vi "PCM Vertical Panel.vi"() -> ()   [LabVIEW 2016, in "PCM PanelSplit.lvclass"]
uses:
  PCM PanelSplit.lvclass
  PanelSplitToolkit/PanelObject/PanelObject.lvclass
  <vilib>/Utility/error.llb/DialogType.ctl
  PanelSplitToolkit/QueueManager.llb/CreatQueue.vi
  PanelSplitToolkit/QueueManager.llb/Remove.vi
  PanelSplitToolkit/QueueManager.llb/Destroy.vi
  PanelSplitToolkit/QueueManager.llb/Insert.vi
  PanelSplitToolkit/PanelDataNode/PanelDataNode.lvclass
  PanelSplitToolkit/PanelDataNode/Split Mode.ctl
panel:
  in  "Node*":refnum<data-value>
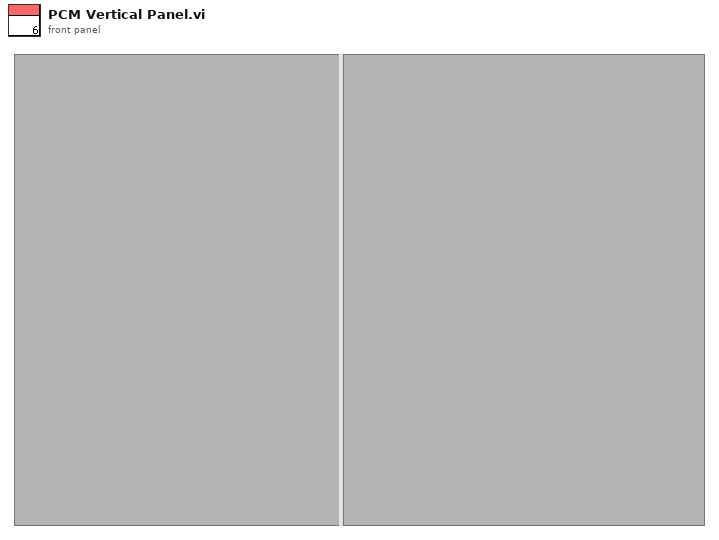
[diagram p1: front panel]
types:
  T1 = cluster{"error":errorcluster, "Event":string, "Data":variant, "Q_Local":string, "Caller":string}
  T2 = typedef "PanelDataNode.lvclass/Split Mode.ctl" = enum16{"Horizontal(up)", "Vertical(left)", "Horizontal(down)", "Vertical(right)"}
  T3 = typedef "DialogType.ctl" = u16
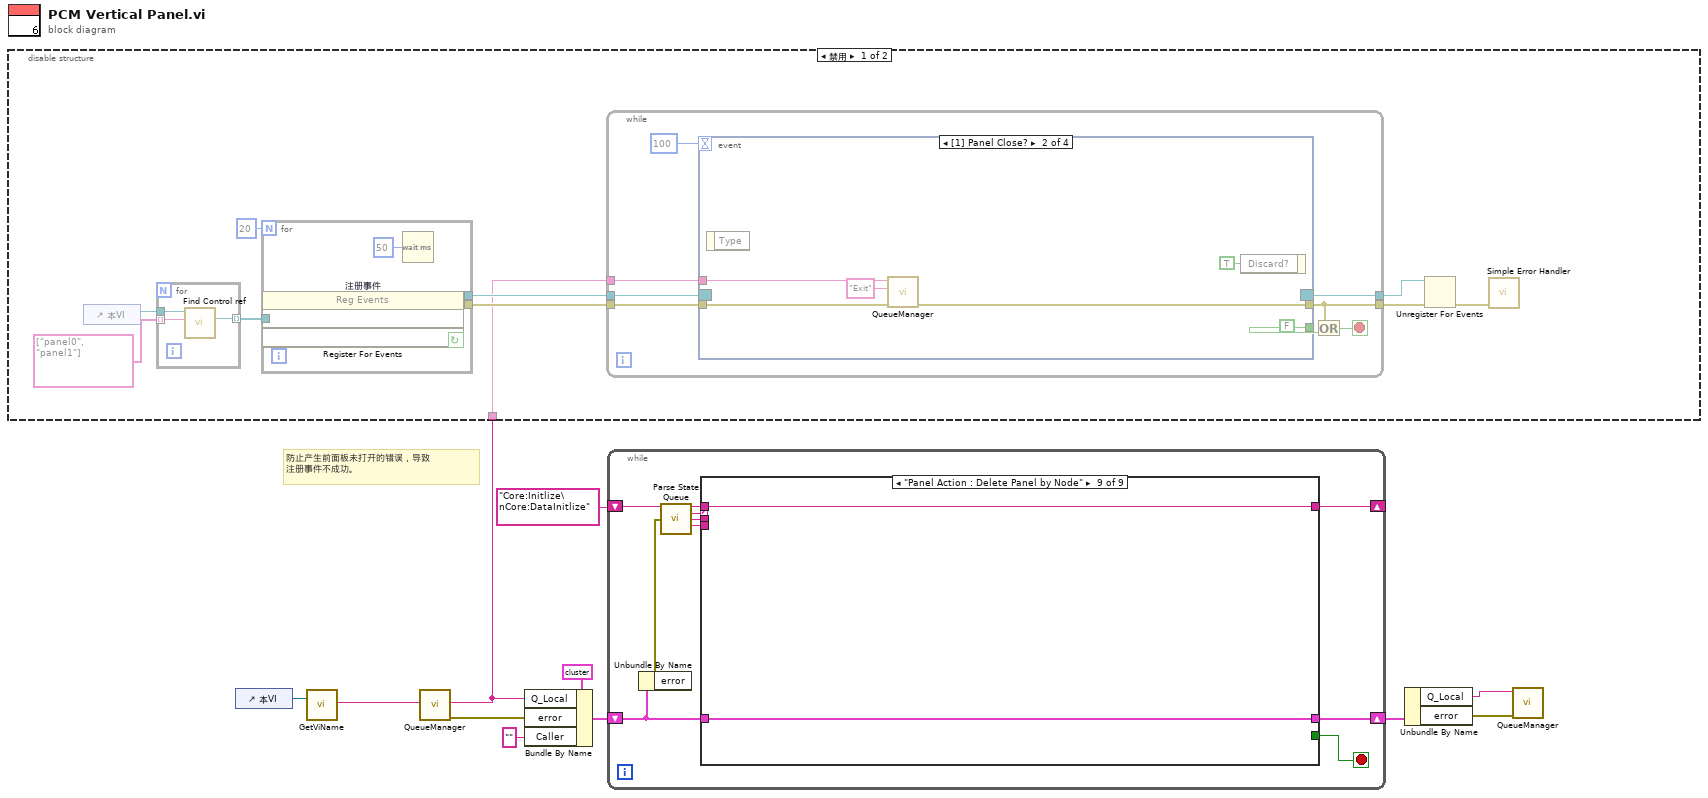
[diagram p0: block diagram]
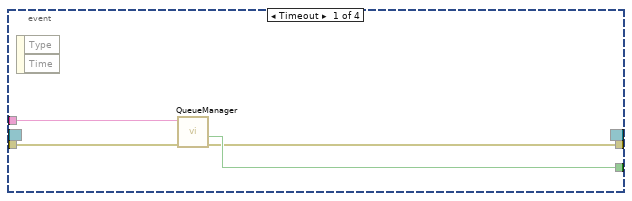
[diagram p2: hidden frame]
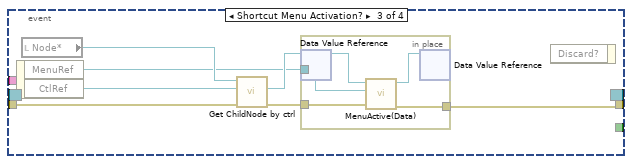
[diagram p3: hidden frame]
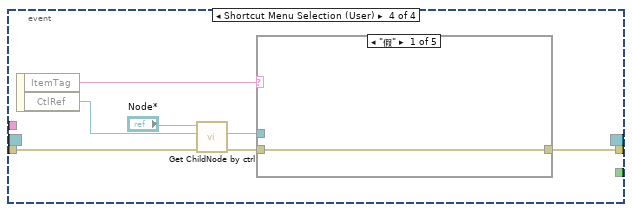
[diagram p4: hidden frame]
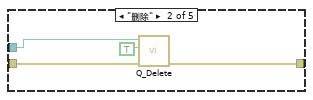
[diagram p5: hidden frame]
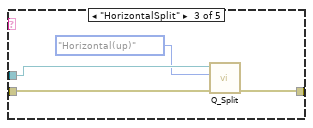
[diagram p6: hidden frame]
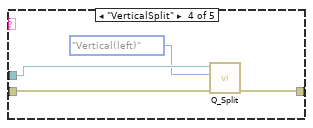
[diagram p7: hidden frame]
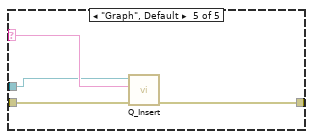
[diagram p8: hidden frame]
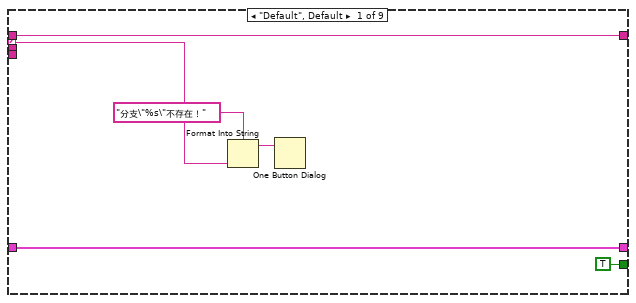
[diagram p10: hidden frame]
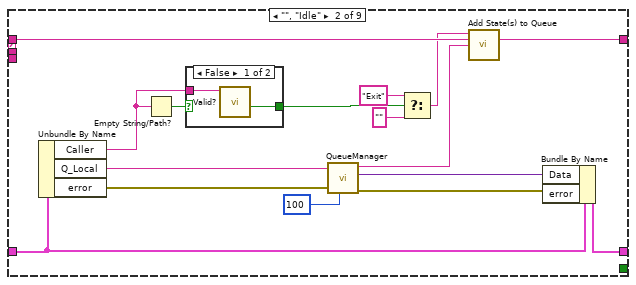
[diagram p11: hidden frame]
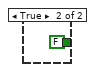
[diagram p12: hidden frame]
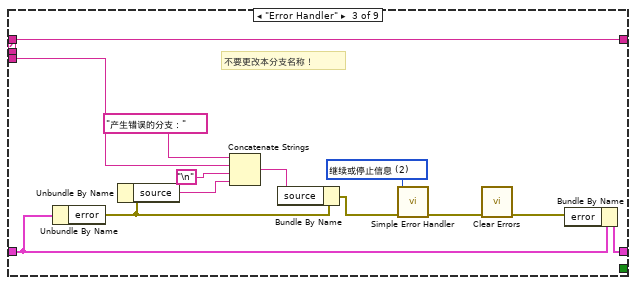
[diagram p13: hidden frame]
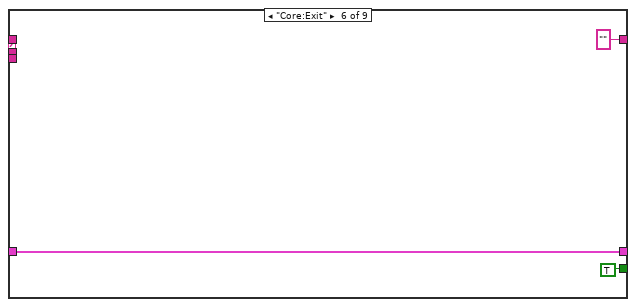
[diagram p16: hidden frame]
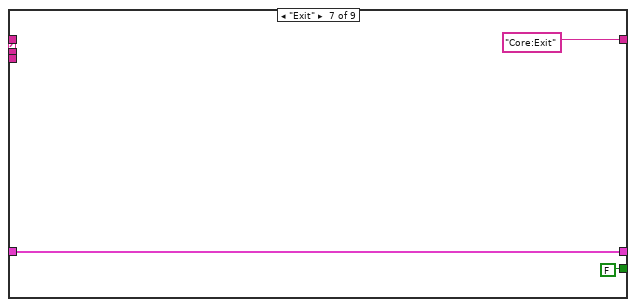
[diagram p17: hidden frame]
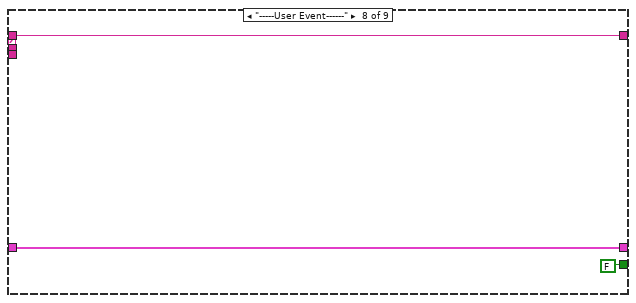
[diagram p18: hidden frame]
diagram:
  # "防止产生前面板未打开的错误，导致\n注册事件不成功。"
  n1 = control-ref of="本VI"() -> (w3:refnum<vi>)
  n2 = call "GetViName.vi"("VI*"=w3) -> ("VI Name"=w1:string)  [unwired: 9 in, 1 out]
  n3 = disable-structure shown="禁用" {
    disable-tunnel: w1 -> [w18 _]
    frame Disabled {
      n4 = control-ref of="本VI"() -> (w12:refnum<vi>)
      n5 = for {
        tunnel: w12 -> [w23]
        tunnel: string[] ["panel0", "panel1"] -> [w22] mode=indexing
        tunnel: [w21] -> w17 mode=indexing
        n6 = call "Find Control ref.vi"("control name"=w22, "panelvi*"=w23) -> ("ctrl*"=w21:refnum<vi>)  [unwired: 7 in, 2 out]
      }
      n7 = for {
        N: 20 -> [_]
        tunnel: [w25] -> w20
        tunnel: [w27] -> w19
        tunnel: w17 -> [w26]
        stop <- w25 continue-if-true
        n8 = register-events "注册事件"(w26, w26) -> (reference out=w27:refnum<event-registration>, error out=w25:errorcluster)  [unwired: 2 in]
        n9 = Wait (ms)(milliseconds to wait=u32 50 ("等待时间（毫秒）")) -> ()  [unwired: 1 out]
      }
      n10 = while {
        tunnel: w20 -> [w29]
        tunnel: w18 -> [w35]
        tunnel: [w32] -> w15
        tunnel: w19 -> [w30]
        tunnel: [w28] -> w13
        stop <- w33 stop-if-true
        n11 = event shown="[1] Panel Close?" {
          selector: w30 -> [_ _ _ _]
          dyn-events: [_ _ _ _] -> w28
          timeout: 100 -> [_ _ _ _]
          tunnel: [w37 FALSE _ _] -> w34
          tunnel: w35 -> [w39 w44 _ _]
          tunnel: w29 -> [w38 w43 w49 w62]
          tunnel: [w36 w42 w47 w60] -> w32
          event Timeout {
            n12 = event-data() -> ()  [unwired: 1 in, 2 out]
            n13 = call-poly "QueueManager.vi"("error in (no error)"=w38, "Queue Name(unamed)"=w39) -> ("error out"=w36:errorcluster, "Not Exist?"=w37:bool)  [unwired: 8 in]
          }
          event Panel Close? {
            n14 = event-data() -> ()  [unwired: 1 in, 1 out]
            n15 = call-poly "QueueManager.vi"("error in"=w43, "Event"="Exit", "QueueName"=w44) -> ("error out"=w42:errorcluster)  [unwired: 7 in, 1 out]
            n16 = event-data("Discard?"=TRUE ("放弃？")) -> ()  [unwired: 1 in, 1 out]
          }
          event Shortcut Menu Activation? {
            n17 = event-data() -> ("MenuRef"=w46:refnum<k9>, "CtlRef"=w50:refnum<vi>)  [unwired: 1 in]
            n18 = local read "Node*"() -> (w51:refnum<data-value>)
            n19 = call "Get ChildNode by ctrl.vi"("error in (no error)"=w49, "ctr*"=w50, "Node*"=w51) -> ("error out"=w48:errorcluster, "ChildNode*"=w52:refnum<data-value>)  [unwired: 7 in]
            n20 = in-place {
              in-place-border: w46 -> [w56]
              in-place-border: w48 -> [w54]
              in-place-border: [w53] -> w47
              n21 = in-place-dvr #1(w52) -> (w57:refnum<class "PanelDataNode.lvclass">)  [unwired: 1 out]
              n22 = call-dynamic "MenuActive(Data).vi"("error in"=w54, "Menu Reference in"=w56, "PanelDataNode in"=w57) -> ("error out"=w53:errorcluster, "PanelDataNode out"=w55:refnum<class "PanelDataNode.lvclass">)  [unwired: 6 in, 1 out]
              n23 = in-place-dvr #1(w55) -> ()  [unwired: 2 out]
            }
            n24 = event-data() -> ()  [unwired: 2 in, 1 out]
          }
          event Shortcut Menu Selection (User) {
            n25 = event-data() -> ("ItemTag"=w59:string, "CtlRef"=w63:refnum<vi>)  [unwired: 1 in]
            n26 = call "Get ChildNode by ctrl.vi"("error in (no error)"=w62, "ctr*"=w63, "Node*"="Node*") -> ("error out"=w61:errorcluster, "ChildNode*"=w58:refnum<data-value>)  [unwired: 7 in]
            n27 = case shown="\"假\"" w59 {
              selector: w59 -> [_ _ _ _ w81]
              tunnel: w61 -> [w65 w68 w73 w77 w80]
              tunnel: [w65 w67 w72 w76 w78] -> w60
              tunnel: w58 -> [_ w66 w71 w75 w79]
              frame "假" {
              }
              frame "删除" {
                n28 = call "Q_Delete.vi"("error in"=w68, "CloseVI?(T)"=TRUE, "ChildNode*"=w66) -> ("error out"=w67:errorcluster)  [unwired: 8 in]
              }
              frame "HorizontalSplit" {
                n29 = call "Q_Split.vi"("error in"=w73, "Split Mode"=Split_Mode."Horizontal(up)", "ChildNode*"=w71) -> ("error out"=w72:errorcluster)  [unwired: 8 in]
              }
              frame "VerticalSplit" {
                n30 = call "Q_Split.vi"("error in"=w77, "Split Mode"=Split_Mode."Vertical(left)", "ChildNode*"=w75) -> ("error out"=w76:errorcluster)  [unwired: 8 in]
              }
              frame "Graph", Default {
                n31 = call "Q_Insert.vi"("error in"=w80, "Vi Alias"=w81, "ChildNode*"=w79) -> ("error out"=w78:errorcluster)  [unwired: 8 in]
              }
            }
          }
        }
        n32 = Or(x=w32, y=w34) -> (x .or. y?=w33:bool)
      }
      n33 = Unregister For Events(event registration refnum=w13, error in=w15) -> (error out=w14:errorcluster)
      n34 = call <vilib>:"Simple Error Handler.vi"("error in (no error)"=w14) -> ()  [unwired: 4 in, 5 out]
    }
    frame Enabled {
    }
  }
  n35 = call-poly "QueueManager.vi"("QueueName"=w1) -> ("error out"=w2:errorcluster)  [unwired: 9 in, 1 out]
  n36 = Bundle By Name(cluster=T1 {"error"={"status"=FALSE, "code"=0, "source"=""}, "Event"="", "Data"=variant, "Q_Local"="", "Caller"=""} ("TmpData"), "Q_Local"=w1, "error"=w2, "Caller"="") -> (w6:T1)
  n37 = while {
    shift-right: [w85] -> w8
    shift-left: w6 -> [w86]
    shift-right: [w84] -> _
    shift-left: "Core:Initlize\nCore:DataInitlize" -> [w91]
    stop <- w88 stop-if-true
    n38 = Unbundle By Name(w86) -> ("error"=w87:errorcluster)
    n39 = call "Parse State Queue.vi"("State Queue"=w91, "Error In (no error)"=w87) -> ("Remaining States"=w90:string, "Current State"=w89:string, "Arguments"=w83:string, "PreState"=w82:string)  [unwired: 10 in]
    n40 = case shown="\"Panel Action : Delete Panel by Node\"" w89 {
      selector: w89 -> [w95 _ _ _ _ _ _ _ _]
      tunnel: w90 -> [w96 w110 w129 w131 w133 _ _ w140 w143]
      tunnel: w83 -> [_ _ _ _ _ _ _ _ _]
      tunnel: [TRUE _ _ _ _ TRUE FALSE FALSE _] -> w88
      tunnel: w86 -> [w97 w107 w126 w130 w132 w135 w138 w141 w144]
      tunnel: [w97 w112 w125 w130 w132 w135 w138 w141 w144] -> w85
      tunnel: [w96 w109 w129 w131 w133 "" ("Remaining States") "Core:Exit" ("Remaining States") w140 w143] -> w84
      tunnel: w82 -> [_ _ w123 _ _ _ _ _ _]
      frame "Default", Default {
        n41 = Format Into String(format string="分支\"%s\"不存在！" ("格式字符串"), w95) -> (resulting string=w94:string)  [unwired: 2 in, 1 out]
        n42 = One Button Dialog(message=w94) -> ()  [unwired: 1 in, 1 out]
      }
      frame "", "Idle" {
        n43 = Unbundle By Name(w107) -> ("Caller"=w101:string, "Q_Local"=w106:string, "error"=w105:errorcluster)
        n44 = Empty String/Path?(string/path=w101) -> (empty?=w104:bool)
        n45 = case shown="False" w104 {
          tunnel: [w115 FALSE ("Not Exist?")] -> w103
          tunnel: w101 -> [w114 _]
          frame False {
            n46 = call "Valid?.vi"("Queue Name(unamed)"=w114) -> ("Not Exist?"=w115:bool)  [unwired: 9 in, 1 out]
          }
          frame True {
          }
        }
        n47 = call-poly "QueueManager.vi"("Time out(-1)"=100, "error in (no error)"=w105, "Queue Name"=w106) -> ("error out"=w113:errorcluster, "Data"=w111:variant, "Event"=w100:string)  [unwired: 5 in, 1 out]
        n48 = Select(t="Exit" ("Event"), s=w103, f="") -> (s? t:f=w98:string)
        n49 = call "Add State(s) to Queue.vi"("State(s) in Front (\"\")"=w98, "State(s) in (\"\")"=w110, "State(s) at Back (\"\")"=w100) -> ("States Out"=w109:string)  [unwired: 12 in]
        n50 = Bundle By Name(cluster=w107, "Data"=w111, "error"=w113) -> (w112:T1)
      }
      frame "Error Handler" {
        w124 = T3 2 items=["无对话框", "确定信息", "继续或停止信息", "确定信息＋警告", "继续/停止+警告"] ("type of dialog (OK msg:1)")
        # "不要更改本分支名称！"
        n51 = Unbundle By Name(w126) -> ("error"=w118:errorcluster)
        n52 = Unbundle By Name(w118) -> ("source"=w121:string)
        n53 = Concatenate Strings("产生错误的分支：" ("字符串"), w123, "\n", w121) -> (w119:string)
        n54 = Bundle By Name(cluster=w118, "source"=w119) -> (w117:errorcluster)
        n55 = call <vilib>:"Simple Error Handler.vi"("type of dialog (OK msg:1)"=w124, "error in (no error)"=w117) -> ("error out"=w127:errorcluster)  [unwired: 3 in, 4 out]
        n56 = call <vilib>:"Clear Errors.vi"("error in (no error)"=w127) -> ("error out"=w128:errorcluster)  [unwired: 5 in, 1 out]
        n57 = Bundle By Name(cluster=w126, "error"=w128) -> (w125:T1)
      }
      frame "Core:Initlize" {
      }
      frame "Core:DataInitlize" {
      }
      frame "Core:Exit" {
      }
      frame "Exit" {
      }
      frame "-----User Event------" {
      }
      frame "Panel Action : Delete Panel by Node" {
      }
    }
  }
  n58 = Unbundle By Name(w8) -> ("Q_Local"=w5:string, "error"=w9:errorcluster)
  n59 = call-poly "QueueManager.vi"("error in (no error)"=w9, "QueeuName"=w5) -> ()  [unwired: 9 in, 1 out]
